vi "Get Dependency State Events.vi"(8 "error in (no error)":errorcluster, 11 "SMO in":refnum<class "SMO.lvclass">) -> (0 "error out":errorcluster, 1 "Error [Dependencies]":refnum<user-event>[](array[refnum]), 2 "State [Dependencies]":refnum<user-event>[](array[refnum]), 3 "SMO out":refnum<class "SMO.lvclass">, 4 "Message [Dependencies]":refnum<user-event>[](array[refnum]), 5 "[Dependencies]":refnum<class "SMO.lvclass">[](array[class]))   [LabVIEW 2019, in "SMO.lvclass"]
doc: "JKI State Machine Objects (SMO) 1.3.0.56\nJKI - JKI\nCopyright (c) 2017, JKI"
uses:
  SMO.lvclass
  Typedefs/SMOState --Enum.ctl
  Support/Attribute.Owner/Packet -- Cluster.ctl
  Support/Attribute.Owner/Attribute.Owner.lvclass
  C:/Users/Patrick/Documents/GitHub/Test (LV2019)/lv-venv/lv.lib/vi.lib/JKI/JKI SMO/Support/Attribute/Attribute.lvclass
  Support/Attribute.Owner/Attribute.Owner.lvclass/Attribute.Owner.ctl
  Support/Attribute/Attribute.lvclass
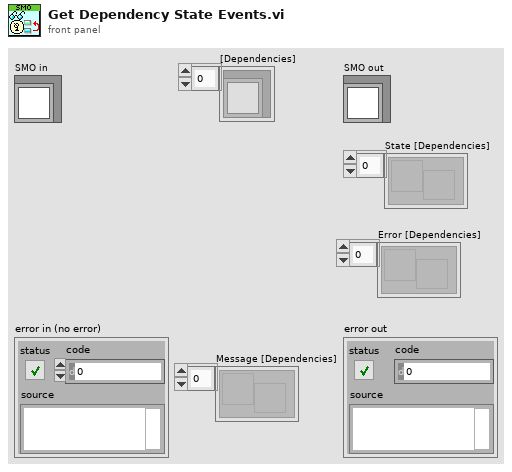
[diagram p1: front panel]
types:
  T1 = typedef "SMO.lvclass/Public Events.ctl" = cluster{"Error":refnum<user-event>, "State":refnum<user-event>, "Reserve State":refnum<user-event>}
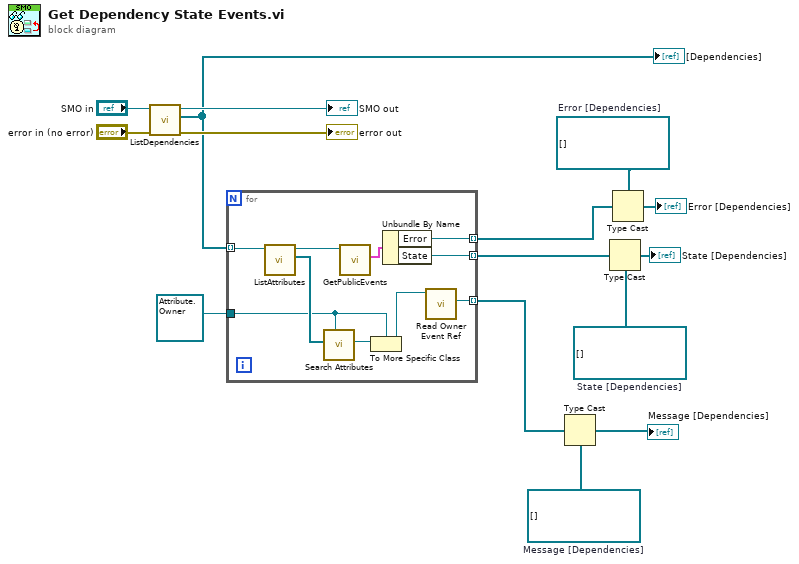
[diagram p0: block diagram]
diagram:
  w4 = refnum<user-event>[] []  # Message [Dependencies]
  w5 = refnum<user-event>[] []  # Error [Dependencies]
  w13 = refnum<user-event>[] [] items=["unknown", "Created", "Started", "Stopped"]  # State [Dependencies]
  n1 = call "ListDependencies.vi"("error in (no error)"="error in (no error)", "SMO in"="SMO in") -> ("error out"=→"error out":errorcluster, "[Dependencies]"=w8:refnum<class "SMO.lvclass">[], "SMO out"=→"SMO out":refnum<class "SMO.lvclass">)  [unwired: 6 in, 1 out]
  "[Dependencies]" <- w8
  n2 = for {
    tunnel: w8 -> [w21] mode=indexing
    tunnel: [w24] -> w14 mode=indexing
    tunnel: [w23] -> w7 mode=indexing
    tunnel: [w22] -> w2 mode=indexing
    tunnel: refnum<class "Attribute.Owner.lvclass"> refnum ("Attribute.Owner.lvclass") -> [w17]
    n3 = call "ListAttributes.vi"("SMO in"=w21) -> ("[Attributes]"=w19:refnum<class "Attribute.lvclass">[], "SMO out"=w20:refnum<class "SMO.lvclass">)  [unwired: 8 in, 1 out]
    n4 = call "Search Attributes.vi"("Attribute type"=w17, "[Attributes]"=w19) -> ("Attribute out"=w18:refnum<class "Attribute.lvclass">)  [unwired: 8 in, 1 out]
    n5 = call "GetPublicEvents.vi"("SMO"=w20) -> ("Public Events"=w25:T1)  [unwired: 8 in, 2 out]
    n6 = To More Specific Class(target class=w17, reference=w18) -> (specific class reference=w16:refnum<class "Attribute.Owner.lvclass">)  [unwired: 1 in, 1 out]
    n7 = Unbundle By Name(w25) -> ("Error"=w23:refnum<user-event>, "State"=w24:refnum<user-event>)
    n8 = call "Read Owner Event Ref.vi"("Attribute.Owner in"=w16) -> ("Upstream Ref"=w22:refnum<user-event>)  [unwired: 8 in, 2 out]
  }
  n9 = Type Cast(type=w4, x=w2) -> (*(type *) &x=→"Message [Dependencies]":refnum<user-event>[])
  n10 = Type Cast(type=w13, x=w14) -> (*(type *) &x=→"State [Dependencies]":refnum<user-event>[])
  n11 = Type Cast(type=w5, x=w7) -> (*(type *) &x=→"Error [Dependencies]":refnum<user-event>[])
